vi "WSVCAP SHL Host TL I2C Write - Multiple Device - Unique Data.vi"(0 "C1 Data":u8[](array[numeric]) format="%.0x", 5 "C2 Data":u8[](array[numeric]) format="%.0x", 7 "C3 Data":u8[](array[numeric]) format="%.0x", 9 "Sub Address":u8=20 format="%.0x", 11 "error in":errorcluster, 12 "Log (T)":bool=TRUE, 13 "DUT Mask Array (All)":bool[][](array[boolean])=[[TRUE, TRUE, TRUE, TRUE, TRUE, TRUE, TRUE, TRUE, TRUE, TRUE, TRUE, TRUE, TRUE, TRUE, TRUE, TRUE, FALSE, FALSE, FALSE, FALSE, FALSE, FALSE, FALSE, FALSE, FALSE, FALSE, FALSE, FALSE, FALSE, FALSE, FALSE, FALSE], [TRUE, TRUE, TRUE, TRUE, TRUE, TRUE, TRUE, TRUE, TRUE, TRUE, TRUE, TRUE, TRUE, TRUE, TRUE, TRUE, FALSE, FALSE, FALSE, FALSE, FALSE, FALSE, FALSE, FALSE, FALSE, FALSE, FALSE, FALSE, FALSE, FALSE, FALSE, FALSE], [TRUE, TRUE, TRUE, TRUE, TRUE, TRUE, TRUE, TRUE, TRUE, TRUE, TRUE, TRUE, TRUE, TRUE, TRUE, TRUE, TRUE, FALSE, FALSE, FALSE, FALSE, FALSE, TRUE, FALSE, FALSE, FALSE, FALSE, FALSE, FALSE, FALSE, FALSE, TRUE], [FALSE, FALSE, FALSE, FALSE, FALSE, FALSE, FALSE, FALSE, FALSE, FALSE, FALSE, FALSE, FALSE, FALSE, FALSE, FALSE, TRUE, FALSE, FALSE, FALSE, FALSE, FALSE, TRUE, FALSE, FALSE, FALSE, FALSE, FALSE, FALSE, FALSE, FALSE, TRUE]], 14 "DUT Mask Mode (All)":T1=enum."All") -> (15 "error out":errorcluster)   [LabVIEW 2012]
uses:
  Type Defs/WSVCAP SHL I2C DUT Mask Mode Enum.ctl
panel:
  out "C3 Data Out":u8[](array[numeric]) format="%.0x"
  out "Socket Mask":u64=1 format="%02x"
  out "C2 Data Out":u8[](array[numeric]) format="%.0x"
  out "C1 Data Out":u8[](array[numeric]) format="%.0x"
  # "DUT 01"
  # "DUT 02"
  # "DUT 03"
  # "DUT 04"
  # "DUT 05"
  # "DUT 06"
  # "DUT 07"
  # "DUT 08"
  # "DUT 09"
  # "DUT 10"
  # "DUT 11"
  # "DUT 12"
  # "DUT 13"
  # "DUT 14"
  # "DUT 15"
  # "DUT 16"
  # "C1"
  # "C2"
  # "C3"
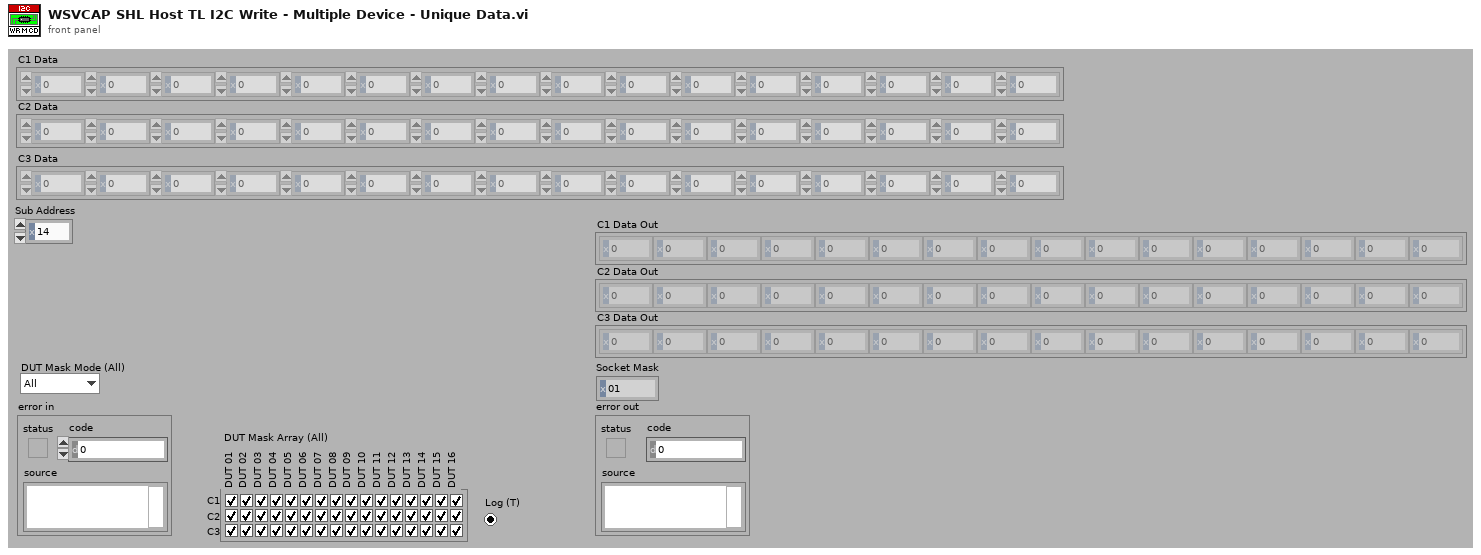
[diagram p1: front panel]
types:
  T1 = typedef "WSVCAP SHL I2C DUT Mask Mode Enum.ctl" = enum16{"Custom", "C1", "C2", "C3", "All"}
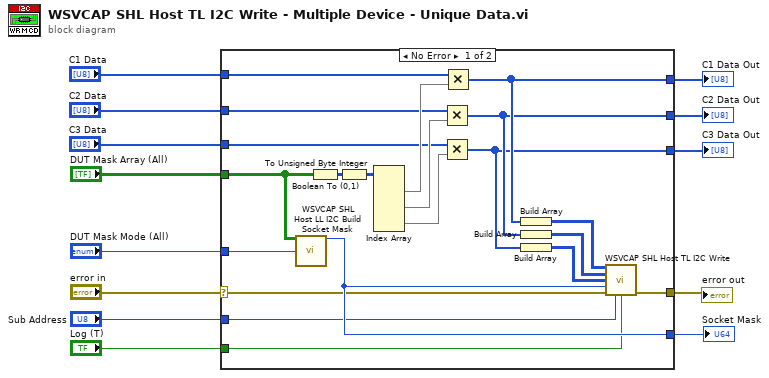
[diagram p0: block diagram]
diagram:
  n1 = case shown="No Error" "error in" {
    selector: "error in" -> [w24 w35]
    tunnel: [w34 w35] -> w13
    tunnel: "Sub Address" -> [w20 _]
    tunnel: [w25 _] -> w10
    tunnel: [w26 _] -> w9
    tunnel: [w31 _] -> w8
    tunnel: "DUT Mask Array (All)" -> [w18 _]
    tunnel: "Log (T)" -> [w23 _]
    tunnel: [w19 _] -> w5
    tunnel: "DUT Mask Mode (All)" -> [w17 _]
    tunnel: "C1 Data" -> [w16 _]
    tunnel: "C2 Data" -> [w15 _]
    tunnel: "C3 Data" -> [w14 _]
    frame No Error {
      n2 = call "WSVCAP SHL Host LL I2C Build Socket Mask.vi"("DUT Mask Array"=w18, "DUT Mask Mode (Custom)"=w17) -> ("Socket Mask [U64]"=w31:u64)  [unwired: 12 in, 1 out]
      n3 = Boolean To (0,1)(Boolean=w18) -> (0, 1=w30:i16[][])
      n4 = To Unsigned Byte Integer(number=w30) -> (unsigned 8bit integer=w27:u8[][])
      n5 = Index Array(array=w27) -> (element #1=w29:u8[], element #2=w28:u8[], element #3=w22:u8[])  [unwired: 6 in]
      n6 = Multiply(x=w15, y=w28) -> (x*y=w25:u8[])
      n7 = Multiply(x=w14, y=w22) -> (x*y=w19:u8[])
      n8 = Multiply(x=w16, y=w29) -> (x*y=w26:u8[])
      n9 = Build Array(w26) -> (w33:u8[][])
      n10 = Build Array(w25) -> (w32:u8[][])
      n11 = Build Array(w19) -> (w21:u8[][])
      n12 = call "WSVCAP SHL Host TL I2C Write.vi"("C1 Data Out"=w33, "C2 Data Out"=w32, "C3 Data Out"=w21, "Socket Mask [U64]"=w31, "error in"=w24, "Sub Address"=w20, "Log (T)"=w23) -> ("error out"=w34:errorcluster)  [unwired: 8 in]
    }
    frame Error {
    }
  }
  "error out" <- w13
  "C1 Data Out" <- w9
  "C2 Data Out" <- w10
  "Socket Mask" <- w8
  "C3 Data Out" <- w5
